vi "RWRHandling_TCP.vi"(0 "TCP Conn":refnum<k5>, 1 "Dictionary":refnum<vi>, 2 "Recieved Data":T1, 3 "H2F Frame":refnum<vi>, 4 "RWR?":bool, 5 "error in (no error)":errorcluster, 6 "SendCmdLED":refnum<vi>, 7 "On/Off Data Ref":refnum<vi>, 8 "RecCmdLED":refnum<vi>, 9 "SensorArr Ref":refnum<vi>) -> (14 "TCP Network Connection out":refnum<k5>, 15 "Bifurcated Recieved Data Out":T1, 16 "Recieved Data":string, 17 "TCP written count":u32, 19 "error out":errorcluster)   [LabVIEW 2018]
doc: "Handles the RWR macro functionality by popping a user prompt asking for User input. This handler uses the TCP/IP Send/Rec VI."
uses:
  TypeDefs/recDataClust.ctl
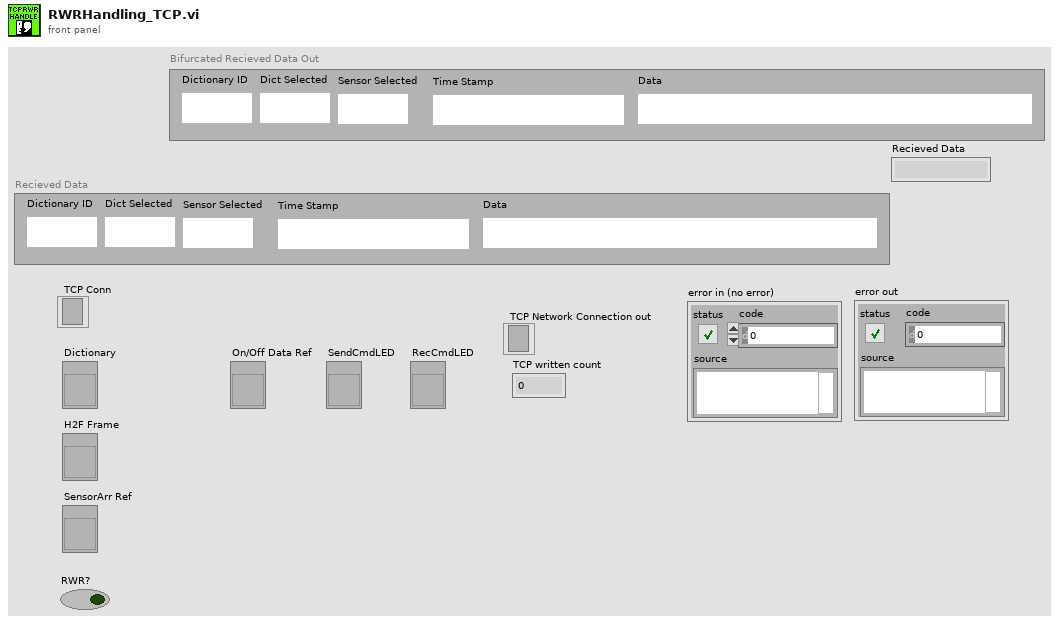
[diagram p1: front panel]
types:
  T1 = typedef "recDataClust.ctl" = cluster{"Dictionary ID":string, "Dict Selected":string, "Sensor Selected":string, "Time Stamp":string, "Data":string}
  T2 = enum32{"No Selection", "WRITE", "READ", "WRITE -> READ", "READ -> WRITE -> READ", "ON/OFF", "NO ARGS"}
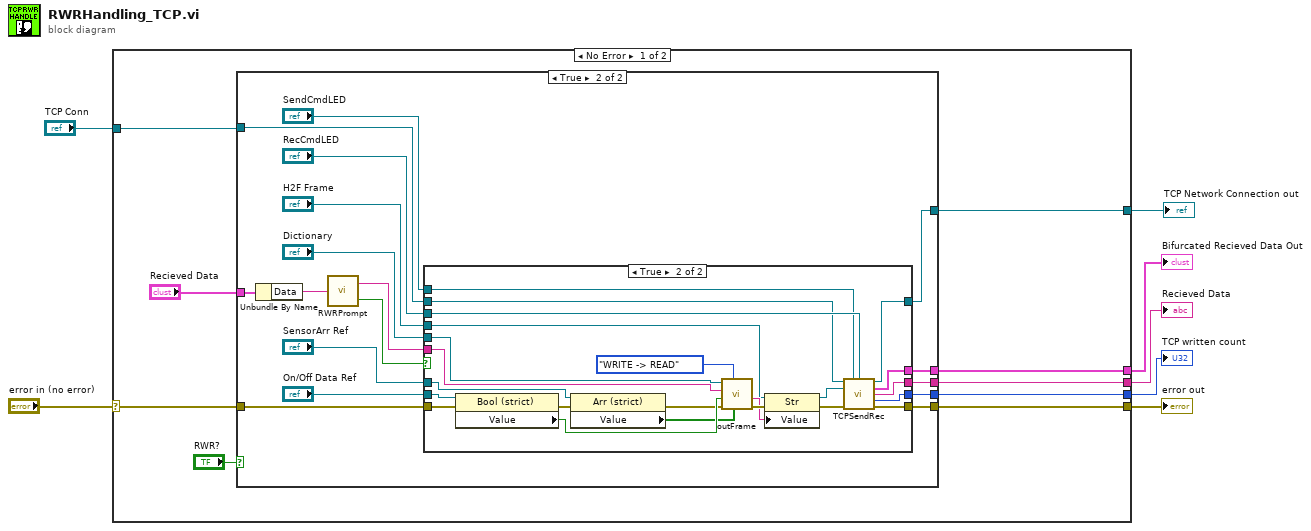
[diagram p0: block diagram]
diagram:
  n1 = case shown="No Error" "error in (no error)" {
    selector: "error in (no error)" -> [w15 w62]
    tunnel: [w16 w62] -> w6
    tunnel: [w12 _] -> w5
    tunnel: [w11 _] -> w4
    tunnel: [w10 _] -> w3
    tunnel: [w9 w61] -> w2
    tunnel: "TCP Conn" -> [w8 w61]
    frame No Error {
      n2 = case shown="True" "RWR?" {
        tunnel: w15 -> [w18 w32]
        tunnel: [w18 w30] -> w16
        tunnel: w8 -> [w17 w29]
        tunnel: "Recieved Data" -> [_ w31]
        tunnel: [w17 w22] -> w9
        tunnel: [_ w21] -> w12
        tunnel: [_ w20] -> w11
        tunnel: [_ w19] -> w10
        frame False {
        }
        frame True {
          n3 = Unbundle By Name(w31) -> ("Data"=w35:string)
          n4 = call "RWRPrompt.vi"("Value Present in Detector 2"=w35) -> ("Value to update in Detector 2"=w33:string, "Cancel Pressed"=w34:bool)
          n5 = case shown="True" w34 {
            tunnel: w33 -> [_ w60]
            tunnel: w32 -> [w37 w56]
            tunnel: [w37 w47] -> w30
            tunnel: w29 -> [w36 w42]
            tunnel: "SensorArr Ref" -> [_ w51]
            tunnel: "Dictionary" -> [_ w50]
            tunnel: "RecCmdLED" -> [_ w44]
            tunnel: "SendCmdLED" -> [_ w43]
            tunnel: "On/Off Data Ref" -> [_ w49]
            tunnel: "H2F Frame" -> [_ w46]
            tunnel: [w36 w41] -> w22
            tunnel: [_ w40] -> w21
            tunnel: [_ w39] -> w20
            tunnel: [_ w38] -> w19
            frame False {
            }
            frame True {
              n6 = property on="Property Node" class="Bool (strict)"(reference=w49, error in=w56) -> (error out=w57:errorcluster, "Value"=w59:bool)  [unwired: 1 out]
              n7 = property on="Property Node" class="Arr (strict)"(reference=w51, error in=w57) -> (error out=w52:errorcluster, "Value"=w58:bool[])  [unwired: 1 out]
              n8 = call "outFrame.vi"("Sensor Array"=w58, "Select Macro Function"=T2."WRITE -> READ", "error in (no error)"=w52, "On/Off Data"=w59, "Write Data (HEX)"=w60, "Cluster in"=w50) -> ("error out"=w54:errorcluster, "H2F Frame"=w53:string)  [unwired: 4 in]
              n9 = property on="Property Node" class="Str"(reference=w46, error in=w54, "Value"=w53) -> (reference out=w45:refnum<vi>, error out=w48:errorcluster)
              n10 = call "TCPSendRec.vi"("TCP Conn"=w42, "SendLEDRef"=w43, "RecLEDRef"=w44, "H2F Frame Ref"=w45, "error in (no error)"=w48) -> ("TCP Network Connection out"=w41:refnum<k5>, "Bifurcated Recieved Data"=w40:T1, "Recieved Frame"=w38:string, "TCP Written Bytes"=w39:i32, "error out"=w47:errorcluster)  [unwired: 6 in]
            }
          }
        }
      }
    }
    frame Error {
    }
  }
  "error out" <- w6
  "TCP written count" <- w4
  "Bifurcated Recieved Data Out" <- w5
  "Recieved Data" <- w3
  "TCP Network Connection out" <- w2
